vi "Set Metadata.vi"(8 "error in (no error)":errorcluster, 10 "Experiment info":T1, 11 "Log Record in":refnum<class "Log Record.lvclass">) -> (0 "error out":errorcluster, 3 "Log Record out":refnum<class "Log Record.lvclass">)   [LabVIEW 2024, in "Log Record.lvclass"]
uses:
  Log Record.lvclass
  NHMFL_Core/Libraries/FAIR Data/MagX/Experiment info.ctl
  Log Record.lvclass/Log Record.ctl
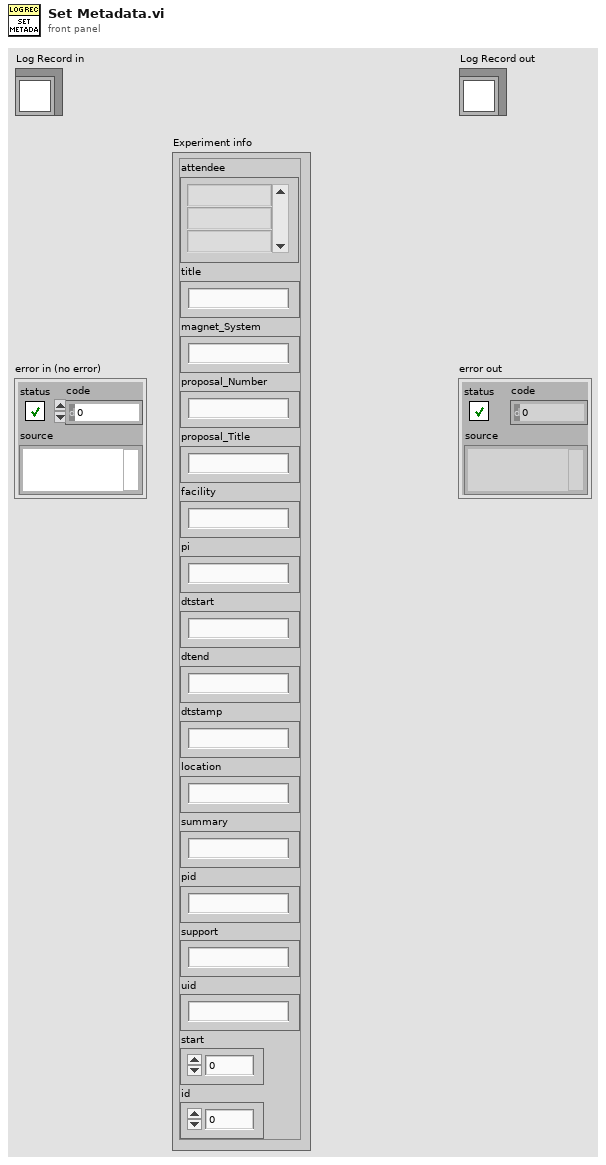
[diagram p1: front panel]
types:
  T1 = typedef "Experiment info.ctl" = cluster{"attendee":string[], "title":string, "magnet_System":string, "proposal_Number":string, "proposal_Title":string, "facility":string, "pi":string, "dtstart":string, "dtend":string, "dtstamp":string, "location":string, "summary":string, "pid":string, "support":string, "uid":string, "start":u64, "id":u64}
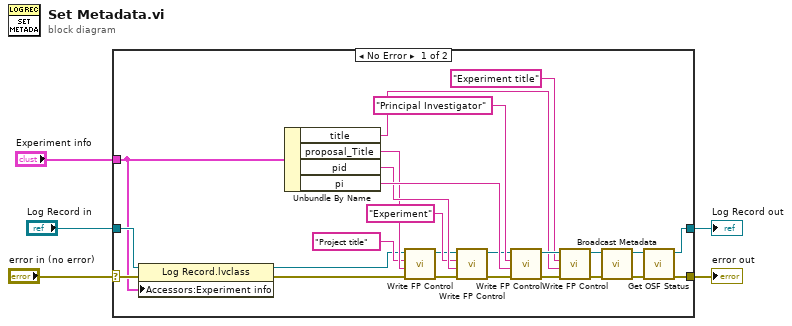
[diagram p0: block diagram]
diagram:
  n1 = case shown="No Error" "error in (no error)" {
    selector: "error in (no error)" -> [w19 w32]
    tunnel: [w11 w32] -> w4
    tunnel: [w12 w31] -> w2
    tunnel: "Log Record in" -> [w30 w31]
    tunnel: "Experiment info" -> [w8 _]
    frame No Error {
      n2 = property class="Log Record.lvclass"(reference=w30, error in=w19, "Accessors:Experiment info"=w8) -> (reference out=w9:refnum<class "Log Record.lvclass">, error out=w10:errorcluster)
      n3 = Unbundle By Name(w8) -> ("title"=w15:string, "proposal_Title"=w21:string, "pid"=w25:string, "pi"=w29:string)
      n4 = call-dynamic "Write FP Control.vi"("error in (no error)"=w10, "Control Value"=w21, "Control Name"="Project title", "Measure Object in"=w9) -> ("error out"=w23:errorcluster, "Measure Object out"=w22:refnum<class "Log Record.lvclass">)  [unwired: 6 in]
      n5 = call-dynamic "Write FP Control.vi"("error in (no error)"=w23, "Control Value"=w25, "Control Name"="Experiment", "Measure Object in"=w22) -> ("error out"=w26:errorcluster, "Measure Object out"=w27:refnum<class "Log Record.lvclass">)  [unwired: 6 in]
      n6 = call-dynamic "Write FP Control.vi"("error in (no error)"=w26, "Control Value"=w29, "Control Name"="Principal Investigator", "Measure Object in"=w27) -> ("error out"=w17:errorcluster, "Measure Object out"=w18:refnum<class "Log Record.lvclass">)  [unwired: 6 in]
      n7 = call-dynamic "Write FP Control.vi"("error in (no error)"=w17, "Control Value"=w15, "Control Name"="Experiment title", "Measure Object in"=w18) -> ("error out"=w7:errorcluster, "Measure Object out"=w6:refnum<class "Log Record.lvclass">)  [unwired: 6 in]
      n8 = call-dynamic "Broadcast Metadata.vi"("error in (no error)"=w7, "Log Record in"=w6) -> ("error out"=w14:errorcluster, "Log Record out"=w13:refnum<class "Log Record.lvclass">)  [unwired: 8 in]
      n9 = call-dynamic "Get OSF Status.vi"("error in (no error)"=w14, "Log Record in"=w13) -> ("error out"=w11:errorcluster, "Log Record out"=w12:refnum<class "Log Record.lvclass">)  [unwired: 7 in, 1 out]
    }
    frame Error {
    }
  }
  "error out" <- w4
  "Log Record out" <- w2
